vi "read-autofocus-file.vi"   [LabVIEW 2014]
uses:
  Start all VIs Globals.vi
  <vilib>/Utility/config.llb/Read Key (Boolean).vi
  TIRF Lock/autofocus-globals.vi
  <vilib>/Utility/config.llb/Read Key (Double).vi
  <vilib>/Utility/config.llb/Read Key (I32).vi
  <vilib>/Utility/config.llb/NI_LVConfig.lvlib
types:
  T1 = enum32{"Invalid", "Standard", "Closed", "Hidden", "Minimized", "Maximized"}
  T2 = typedef "NI_LVConfig.lvlib/Config Data RefNum.ctl" = refnum<k1>
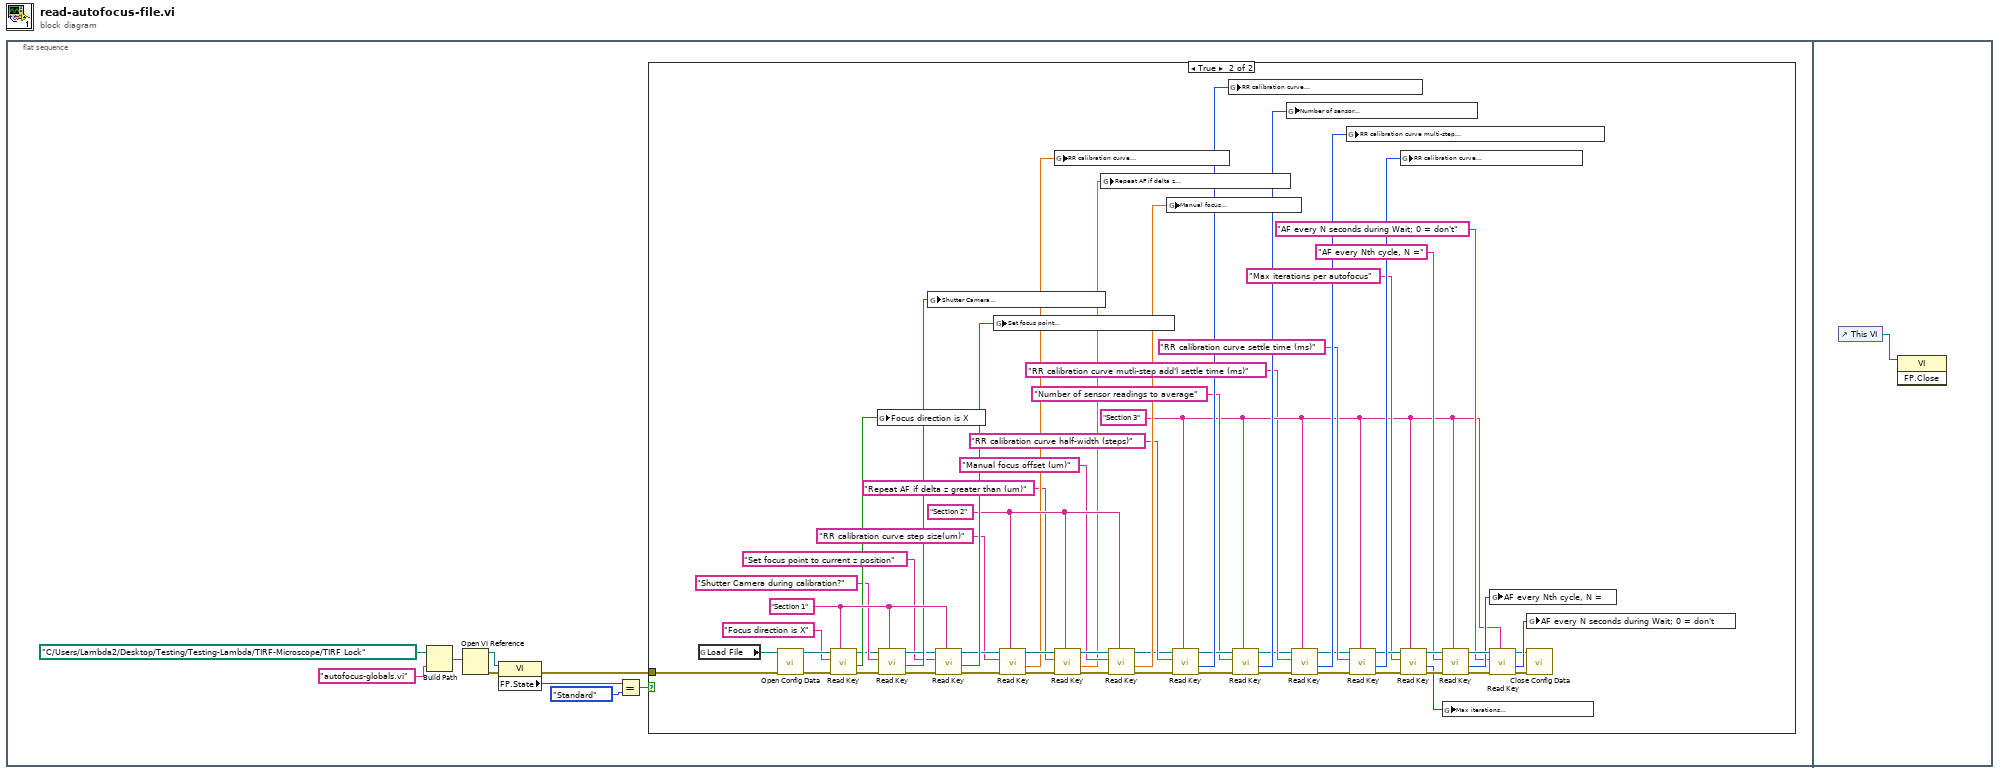
[diagram p0: block diagram]
diagram:
  n1 = flat-sequence {
    frame #0 {
      n2 = Build Path(base path=path "C:/Users/Lambda2/Desktop/Testing/Testing-Lambda/TIRF-Microscope/TIRF Lock", name or relative path="autofocus-globals.vi") -> (appended path=w9:path)
      n3 = Open VI Reference(vi path=w9) -> (vi reference=w8:refnum<vi>, error out=w7:errorcluster)  [unwired: 1 in, 4 out]
      n4 = property class="VI"(reference=w8, error in=w7) -> (error out=w3:errorcluster, "FP.State"=w4:T1)  [unwired: 1 out]
      n5 = Equal?(x=w4, y=T1."Standard") -> (x = y?=w2:bool)
      n6 = case shown="True" w2 {
        tunnel: w3 -> [_ w68]
        frame False {
        }
        frame True {
          w13 = "Section 3"
          w48 = "Section 2"
          w63 = "Section 1"
          n7 = global read "Start all VIs Globals.vi" "Load File"() -> (w19:path)
          n8 = call <vilib>:"Open Config Data.vi"("error in (no error)"=w68, "configuration file path"=w19) -> ("error out"=w67:errorcluster, "refnum"=w66:T2)  [unwired: 7 in, 1 out]
          n9 = call-poly <vilib>:"Read Key.vi"("section"=w63, "error in (no error)"=w67, "key"="Focus direction is X", "refnum"=w66) -> ("error out"=w65:errorcluster, "value"=w62:bool, "refnum out"=w57:T2)  [unwired: 1 in, 4 out]
          n10 = global write "autofocus-globals.vi" "Focus direction is X"(w62) -> ()
          n11 = call-poly <vilib>:"Read Key.vi"("section"=w63, "error in (no error)"=w65, "key"="Shutter Camera during calibration?", "refnum"=w57) -> ("error out"=w64:errorcluster, "value"=w61:bool, "refnum out"=w56:T2)  [unwired: 1 in, 4 out]
          n12 = global write "autofocus-globals.vi" "Shutter Camera\nduring calibration?"(w61) -> ()
          n13 = call-poly <vilib>:"Read Key.vi"("section"=w63, "error in (no error)"=w64, "key"="Set focus point to current z position", "refnum"=w56) -> ("error out"=w54:errorcluster, "value"=w60:bool, "refnum out"=w53:T2)  [unwired: 1 in, 4 out]
          n14 = global write "autofocus-globals.vi" "Set focus point\nto current z position"(w60) -> ()
          n15 = call-poly <vilib>:"Read Key.vi"("section"=w48, "error in (no error)"=w54, "key"="RR calibration curve step size(um)", "refnum"=w53) -> ("error out"=w52:errorcluster, "value"=w44:dbl, "refnum out"=w51:T2)  [unwired: 1 in, 4 out]
          n16 = global write "autofocus-globals.vi" "RR calibration curve\nstep size (um)"(w44) -> ()
          n17 = call-poly <vilib>:"Read Key.vi"("section"=w48, "error in (no error)"=w52, "key"="Repeat AF if delta z greater than (um)", "refnum"=w51) -> ("error out"=w50:errorcluster, "value"=w42:dbl, "refnum out"=w49:T2)  [unwired: 1 in, 4 out]
          n18 = global write "autofocus-globals.vi" "Repeat AF if delta z \ngreater than (um)"(w42) -> ()
          n19 = call-poly <vilib>:"Read Key.vi"("section"=w48, "error in (no error)"=w50, "key"="Manual focus offset (um)", "refnum"=w49) -> ("error out"=w41:errorcluster, "value"=w47:dbl, "refnum out"=w32:T2)  [unwired: 1 in, 4 out]
          n20 = global write "autofocus-globals.vi" "Manual focus\noffset (um)"(w47) -> ()
          n21 = call-poly <vilib>:"Read Key.vi"("section"=w13, "error in (no error)"=w41, "key"="RR calibration curve half-width (steps)", "refnum"=w32) -> ("error out"=w40:errorcluster, "value"=w35:i32, "refnum out"=w31:T2)  [unwired: 4 in, 1 out]
          n22 = global write "autofocus-globals.vi" "RR calibration curve\nhalf-width  (steps)"(w35) -> ()
          n23 = call-poly <vilib>:"Read Key.vi"("section"=w13, "error in (no error)"=w40, "key"="Number of sensor readings to average", "refnum"=w31) -> ("error out"=w17:errorcluster, "value"=w34:i32, "refnum out"=w11:T2)  [unwired: 4 in, 1 out]
          n24 = global write "autofocus-globals.vi" "Number of sensor\nreadings to average"(w34) -> ()
          n25 = call-poly <vilib>:"Read Key.vi"("section"=w13, "error in (no error)"=w17, "key"="RR calibration curve mutli-step add'l settle time (ms)", "refnum"=w11) -> ("error out"=w16:errorcluster, "value"=w18:i32, "refnum out"=w10:T2)  [unwired: 4 in, 1 out]
          n26 = global write "autofocus-globals.vi" "RR calibration curve multi-step\nadd'l settle time (ms)"(w18) -> ()
          n27 = call-poly <vilib>:"Read Key.vi"("section"=w13, "error in (no error)"=w16, "key"="RR calibration curve settle time (ms)", "refnum"=w10) -> ("error out"=w39:errorcluster, "value"=w33:i32, "refnum out"=w30:T2)  [unwired: 4 in, 1 out]
          n28 = global write "autofocus-globals.vi" "RR calibration curve\nsettle time (ms)"(w33) -> ()
          n29 = call-poly <vilib>:"Read Key.vi"("section"=w13, "error in (no error)"=w39, "key"="Max iterations per autofocus", "refnum"=w30) -> ("error out"=w38:errorcluster, "value"=w27:i32, "refnum out"=w29:T2)  [unwired: 4 in, 1 out]
          n30 = call-poly <vilib>:"Read Key.vi"("section"=w13, "error in (no error)"=w38, "key"="AF every Nth cycle, N =", "refnum"=w29) -> ("error out"=w37:errorcluster, "value"=w25:i32, "refnum out"=w28:T2)  [unwired: 4 in, 1 out]
          n31 = global write "autofocus-globals.vi" "Max iterations \nper autofocus"(w27) -> ()
          n32 = global write "autofocus-globals.vi" "AF every Nth cycle, N ="(w25) -> ()
          n33 = call-poly <vilib>:"Read Key.vi"("section"=w13, "error in (no error)"=w37, "key"="AF every N seconds during Wait; 0 = don't", "refnum"=w28) -> ("error out"=w21:errorcluster, "value"=w24:i32, "refnum out"=w20:T2)  [unwired: 4 in, 1 out]
          n34 = global write "autofocus-globals.vi" "AF every N seconds during Wait; 0 = don't"(w24) -> ()
          n35 = call <vilib>:"Close Config Data.vi"("error in (no error)"=w21, "refnum"=w20) -> ()  [unwired: 1 in, 9 out]
        }
      }
    }
    frame #1 {
      n36 = control-ref of="This VI"() -> (w69:refnum<vi>)
      n37 = invoke class="VI" method="FP.Close"(reference=w69) -> ()  [unwired: 2 in, 3 out]
    }
  }
